vi "Agilent VNA Read Calibration Status.vi"(7 "Agilent VNA":T6, 8 "error in (no error)":errorcluster, 10 "Parameters to Measure":T2[](array[typedef]) {"Channel" min=1 max=99 step=1; "Parameter"."Stimulus Port" min=1 step=1; "Parameter"."Response Port" min=1 step=1}, 11 "VISA Resource Name":refnum<visa-resource-name>) -> (0 "error out":errorcluster {"code" format="%.0x"}, 1 "Parameters to Measure":T2[](array[typedef]) {"Channel" min=1 max=99 step=1; "Parameter"."Stimulus Port" min=1 step=1; "Parameter"."Response Port" min=1 step=1}, 2 "Calibration Type by Parameter":T1[](array[typedef]), 3 "dup VISA Resource Name":refnum<visa-resource-name>)   [LabVIEW 2011]
doc: "This VI for the HP 8753B is used to read the calibration type.\n\n0 response\n1 response and isolation\n2 S11 1-port\n3 S22 1-port\n4 full 2-port\n5 one path 2-port\n6 no cal detected"
uses:
  TypeDefs/Agilent VNA Instrument Info.ctl
  tests/S Parameter/TypeDefs/SP Parameter to Measure.ctl
  tests/S Parameter/TypeDefs/SP Parameter.ctl
  tests/S Parameter/TypeDefs/SP Calibration State.ctl
  tests/S Parameter/TypeDefs/SP Measurement Format.ctl
  TypeDefs/Agilent VNA Calibration State.ctl
  TypeDefs/Agilent VNA Measurement.ctl
  TypeDefs/Agilent VNA Conversion.ctl
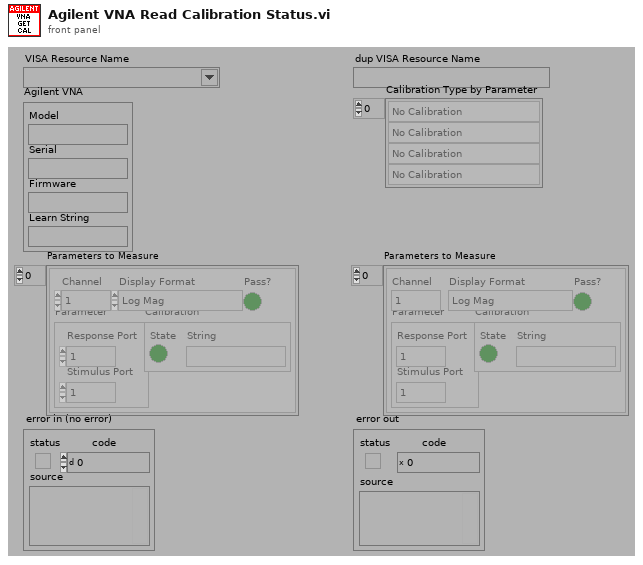
[diagram p1: front panel]
types:
  T1 = typedef "Agilent VNA Calibration State.ctl" = enum32{"No Calibration", "Response", "Response and Isolation", "Full 1-Port (Port 1)", "Full 1-Port (Port 2)", "Full 2-Port", "One Path 2-Port", "TRL/LRM  2-Port", "TOSM Multi-Port", "TOM 2-Port", "TRM 2-Port", "TNA 2-Port", "Full 1-Port (Port 3)", "Full 1-Port (Port 4)", "Full 3-Port", "Full 4-Port", "Full 1-Port (Port 5)", "Full 1-Port (Port 6)", "Full 1-Port (Port 7)", "Full 1-Port (Port 8)", "Full 5-Port", "Full 6-Port", "Full 7-Port", "Full 8-Port"}
  T2 = typedef "SP Parameter to Measure.ctl" = cluster{"Channel":i8, "Parameter":T3, "Calibration":T4, "Display Format":T5, "Pass?":bool}
  T3 = typedef "SP Parameter.ctl" = cluster{"Stimulus Port":i8, "Response Port":i8}
  T4 = typedef "SP Calibration State.ctl" = cluster{"State":bool, "String":string}
  T5 = typedef "SP Measurement Format.ctl" = enum32{"Log Mag", "Phase", "Delay", "Smith (R+jX)", "Polar (Re/Im)", "Linear Mag", "SWR", "Real", "Imaginary", "Smith (Lin/Phase)", "Smith (Log/Phase)", "Smith (Real/Imag)", "Smith (G+jB)", "Polar (Lin/Phase)", "Polar (Log/Phase)", "Expanded Phase", "Positive Phase", "Inverted Smith", "Unwrapped Phase", "Power Out", "Power In", "Linear Mag/Phase", "Log Mag/Phase", "Real/Imaginary"}
  T6 = typedef "Agilent VNA Instrument Info.ctl" = cluster{"Model":string, "Serial":string, "Firmware":string, "Learn String":string}
  T7 = typedef "Agilent VNA Model.ctl" = enum16{"Not Supported", "8510X", "8719X", "8720X", "8722X", "8753X", "ENA", "PNA", "Field Fox"}
  T8 = typedef "Agilent VNA Measurement.ctl" = enum32{"SXX", "Analog In - Aux In", "A/R", "B/R", "A/B", "A", "B", "R"}
  T9 = typedef "Agilent VNA Conversion.ctl" = enum16{"Off", "Z Reflection", "Z Transmit", "Y Reflection", "Y Transmit", "Inversion", "ZT Shunt", "YT Shunt", "Conjugation"}
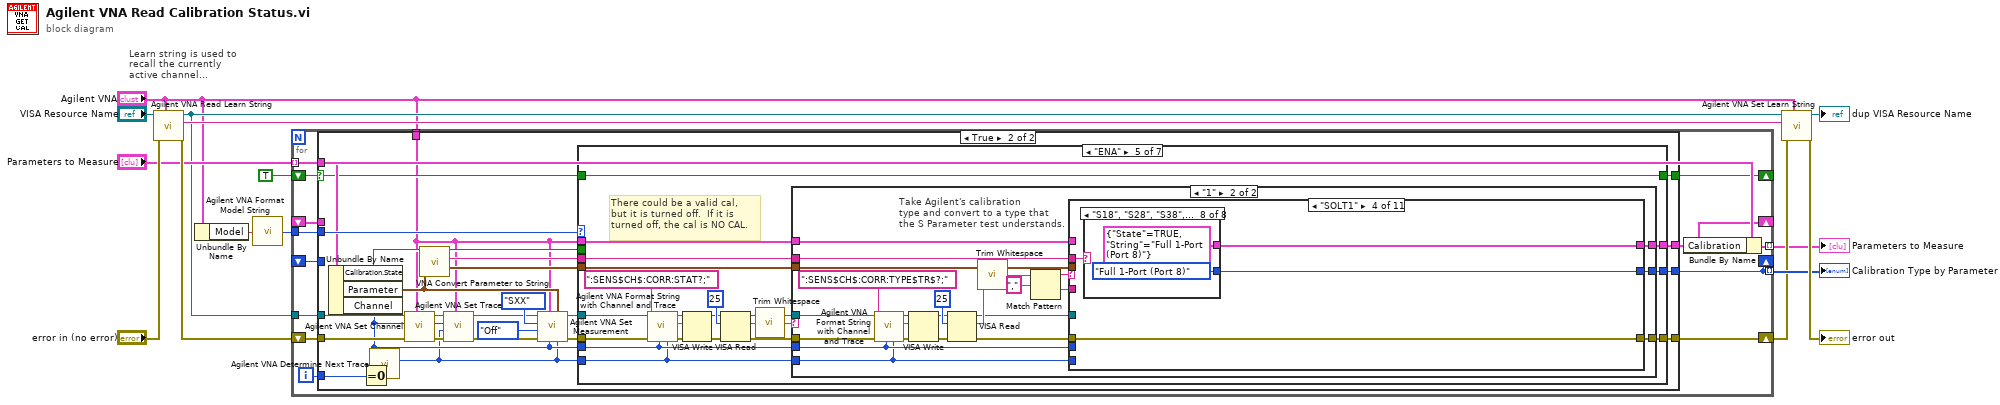
[diagram p0: block diagram]
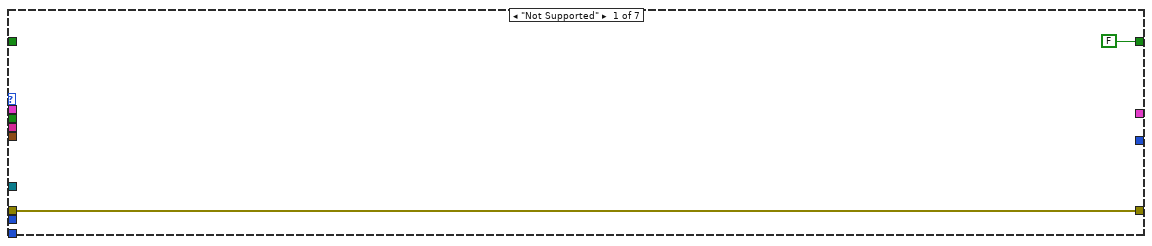
[diagram p3: hidden frame]
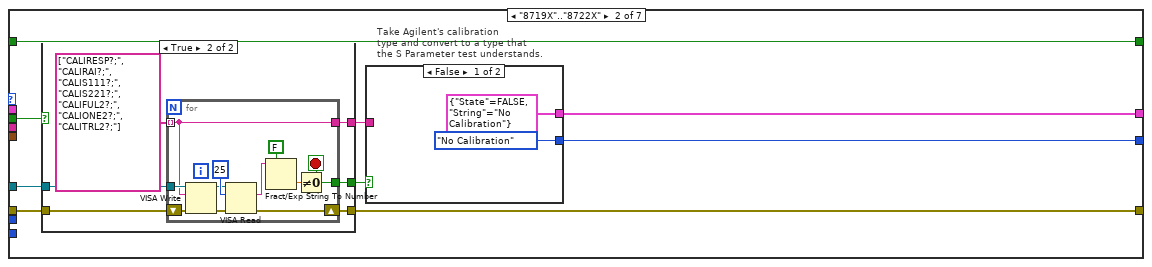
[diagram p4: hidden frame]
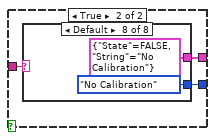
[diagram p6: hidden frame]
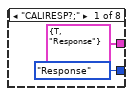
[diagram p7: hidden frame]
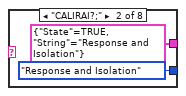
[diagram p8: hidden frame]
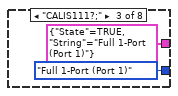
[diagram p9: hidden frame]
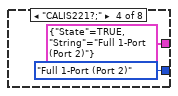
[diagram p10: hidden frame]
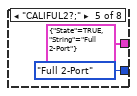
[diagram p11: hidden frame]
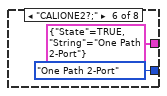
[diagram p12: hidden frame]
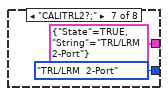
[diagram p13: hidden frame]
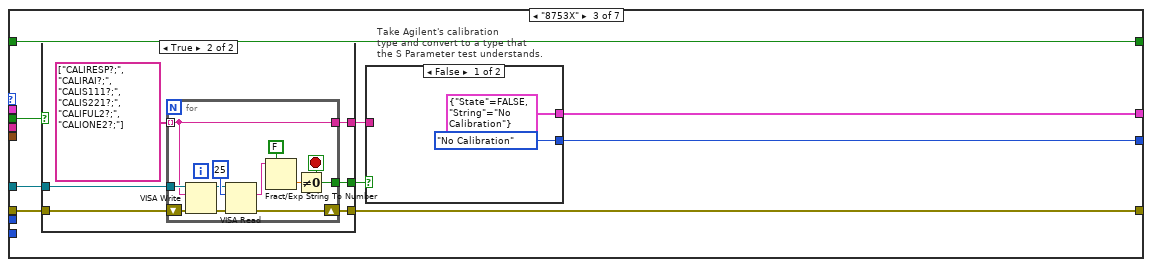
[diagram p14: hidden frame]
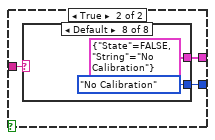
[diagram p16: hidden frame]
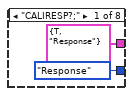
[diagram p17: hidden frame]
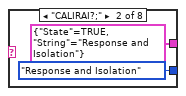
[diagram p18: hidden frame]
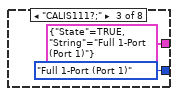
[diagram p19: hidden frame]
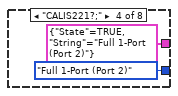
[diagram p20: hidden frame]
diagram:
  # "Learn string is used to\nrecall the currently \nactive channel..."
  n1 = call "Agilent VNA Read Learn String.vi"("Agilent VNA"="Agilent VNA", "error in (no error)"="error in (no error)", "VISA Resource Name"="VISA Resource Name") -> ("error out"=w8:errorcluster, "Learn String"=w13:string, "dup VISA Resource Name"=w6:refnum<visa-resource-name>)  [unwired: 6 out]
  n2 = Unbundle By Name("Agilent VNA") -> ("Model"=w4:string)
  n3 = call "Agilent VNA Format Model String.vi"("Model"=w4) -> ("Model"=w5:T7)
  n4 = for {
    tunnel: w6 -> [w28]
    shift-right: [w29] -> w9
    shift-left: w8 -> [w27]
    tunnel: "Parameters to Measure" -> [w24] mode=indexing
    tunnel: [w18] -> w10 mode=indexing
    tunnel: w5 -> [w25]
    tunnel: [w23] -> w3 mode=indexing
    shift-right: [w22] -> _
    shift-left: TRUE -> [w21]
    tunnel: "Agilent VNA" -> [w20]
    shift-right: [w19] -> _
    shift-left: _ -> [w16]
    shift-right: [w18] -> _
    shift-left: _ -> [w17]
    i -> [w26]
    n5 = case shown="True" w21 {
      selector: w21 -> [w32 w35]
      tunnel: [w33 w56] -> w29
      tunnel: w28 -> [_ w55]
      tunnel: w27 -> [w33 w54]
      tunnel: [w31 w50] -> w18
      tunnel: w26 -> [_ w41]
      tunnel: w25 -> [_ w39]
      tunnel: w24 -> [_ w38]
      tunnel: [w30 w37] -> w19
      tunnel: [w32 w36] -> w22
      tunnel: w20 -> [_ w34]
      tunnel: w17 -> [w31 _]
      tunnel: w16 -> [w30 _]
      frame False {
        # "Do not check subsequent channels and traces.\nJust duplicate the calibration."
      }
      frame True {
        n6 = Unbundle By Name(w38) -> ("Calibration.State"=w53:bool, "Parameter"=w48:T3, "Channel"=w43:i8)
        n7 = Equal To 0?(x=w41) -> (x = 0?=w40:bool)
        n8 = call "Agilent VNA Determine Next Trace.vi"("Reset?"=w40, "Channel"=w43) -> ("Next Trace"=w42:i8)  [unwired: 9 out]
        n9 = call "Agilent VNA Set Channel.vi"("Agilent VNA"=w34, "error in (no error)"=w54, "Channel"=w43, "VISA Resource Name"=w55) -> ("error out"=w47:errorcluster, "dup VISA Resource Name"=w46:refnum<visa-resource-name>)  [unwired: 6 out]
        n10 = call "VNA Convert Parameter to String.vi"("Parameter"=w48) -> ("Parameter String"=w51:string)  [unwired: 10 out]
        n11 = call "Agilent VNA Set Trace.vi"("Agilent VNA"=w34, "error in (no error)"=w47, "Trace"=w42, "Channel"=w43, "VISA Resource Name"=w46) -> ("error out"=w44:errorcluster, "dup VISA Resource Name"=w45:refnum<visa-resource-name>)  [unwired: 5 out]
        n12 = call "Agilent VNA Set Measurement.vi"("Trace"=w42, "Parameter"=w48, "Channel"=w43, "Agilent VNA"=w34, "error in (no error)"=w44, "Conversion (Off)"=Agilent_VNA_Conversion."Off", "Measurement (SXX)"=Agilent_VNA_Measurement."SXX" ("Measurement (S11 - A/R)"), "VISA Resource Name"=w45) -> ("error out"=w58:errorcluster, "dup VISA Resource Name"=w57:refnum<visa-resource-name>)  [unwired: 2 out]
        n13 = case shown="\"ENA\"" w39 {
          tunnel: w58 -> [w60 w69 w117 w174 w217 w344 w435]
          tunnel: w57 -> [_ w68 w116 w173 w212 w339 w433]
          tunnel: [w60 w67 w115 w169 w223 w349 w443] -> w56
          tunnel: [_ w66 w114 w167 w225 w351 w445] -> w50
          tunnel: w53 -> [_ w63 w111 _ _ _ _]
          tunnel: w43 -> [_ _ _ _ w210 w338 w429]
          tunnel: w51 -> [_ _ _ _ w224 w350 w444]
          tunnel: w34 -> [_ _ _ _ w222 w348 _]
          tunnel: [_ w62 w110 w159 w221 w347 w442] -> w37
          tunnel: w42 -> [_ _ _ _ w209 w337 w430]
          tunnel: w48 -> [_ _ _ _ w220 w346 _]
          tunnel: [FALSE w61 w109 w157 w206 FALSE w428] -> w36
          tunnel: w35 -> [_ w61 w109 w157 w206 _ w428]
          frame "Not Supported" {
          }
          frame "8719X".."8722X" {
            # "Take Agilent's calibration\ntype and convert to a type that\nthe S Parameter test understands."
            n14 = case shown="True" w63 {
              tunnel: w69 -> [w70 w76]
              tunnel: w68 -> [_ w75]
              tunnel: [w70 w74] -> w67
              tunnel: [_ w73] -> w65
              tunnel: [_ w72] -> w64
              frame False {
              }
              frame True {
                n15 = for {
                  tunnel: w75 -> [w86]
                  tunnel: [w77] -> w73
                  tunnel: [w78] -> w72
                  shift-right: [w85] -> w74
                  shift-left: w76 -> [w87]
                  tunnel: string[] ["CALIRESP?;", "CALIRAI?;", "CALIS111?;", "CALIS221?;", "CALIFUL2?;", "CALIONE2?;", "CALITRL2?;"] -> [w78] mode=indexing
                  stop <- w77 stop-if-true
                  n16 = VISA Write(VISA resource name=w86, write buffer=w78, error in (no error)=w87) -> (VISA resource name out=w80:refnum<visa-resource-name>, error out=w84:errorcluster)  [unwired: 1 out]
                  n17 = VISA Read(VISA resource name=w80, byte count=u32 25, error in (no error)=w84) -> (read buffer=w83:string, error out=w85:errorcluster)  [unwired: 2 out]
                  n18 = Fract/Exp String To Number(use system decimal point (T)=FALSE, string=w83) -> (number=w82:dbl)  [unwired: 3 out]
                  n19 = Not Equal To 0?(x=w82) -> (x != 0?=w77:bool)
                }
              }
            }
            n20 = case shown="False" w65 {
              tunnel: [Agilent_VNA_Calibration_State."No Calibration" ("S Parameter Test Cal Type") w92] -> w66
              tunnel: w64 -> [_ w91]
              tunnel: [T4 {"State"=FALSE, "String"="No Calibration"} w90] -> w62
              frame False {
              }
              frame True {
                n21 = case shown="Default" w91 {
                  tunnel: [Agilent_VNA_Calibration_State."Response" ("S Parameter Test Cal Type") Agilent_VNA_Calibration_State."Response and Isolation" ("S Parameter Test Cal Type") Agilent_VNA_Calibration_State."Full 1-Port (Port 1)" ("S Parameter Test Cal Type") Agilent_VNA_Calibration_State."Full 1-Port (Port 2)" ("S Parameter Test Cal Type") Agilent_VNA_Calibration_State."Full 2-Port" ("S Parameter Test Cal Type") Agilent_VNA_Calibration_State."One Path 2-Port" ("S Parameter Test Cal Type") Agilent_VNA_Calibration_State."TRL/LRM  2-Port" ("S Parameter Test Cal Type") Agilent_VNA_Calibration_State."No Calibration" ("S Parameter Test Cal Type")] -> w92
                  tunnel: [T4 {"State"=TRUE, "String"="Response"} T4 {"State"=TRUE, "String"="Response and Isolation"} T4 {"State"=TRUE, "String"="Full 1-Port (Port 1)"} T4 {"State"=TRUE, "String"="Full 1-Port (Port 2)"} T4 {"State"=TRUE, "String"="Full 2-Port"} T4 {"State"=TRUE, "String"="One Path 2-Port"} T4 {"State"=TRUE, "String"="TRL/LRM 2-Port"} T4 {"State"=FALSE, "String"="No Calibration"}] -> w90
                  frame "CALIRESP?;" {
                  }
                  frame "CALIRAI?;" {
                  }
                  frame "CALIS111?;" {
                  }
                  frame "CALIS221?;" {
                  }
                  frame "CALIFUL2?;" {
                  }
                  frame "CALIONE2?;" {
                  }
                  frame "CALITRL2?;" {
                  }
                  frame Default {
                  }
                }
              }
            }
          }
          frame "8753X" {
            # "Take Agilent's calibration\ntype and convert to a type that\nthe S Parameter test understands."
            n22 = case shown="True" w111 {
              tunnel: w117 -> [w118 w124]
              tunnel: w116 -> [_ w123]
              tunnel: [w118 w122] -> w115
              tunnel: [_ w121] -> w113
              tunnel: [_ w120] -> w112
              frame False {
              }
              frame True {
                n23 = for {
                  tunnel: w123 -> [w134]
                  tunnel: [w125] -> w121
                  tunnel: [w126] -> w120
                  shift-right: [w133] -> w122
                  shift-left: w124 -> [w135]
                  tunnel: string[] ["CALIRESP?;", "CALIRAI?;", "CALIS111?;", "CALIS221?;", "CALIFUL2?;", "CALIONE2?;"] -> [w126] mode=indexing
                  stop <- w125 stop-if-true
                  n24 = VISA Write(VISA resource name=w134, write buffer=w126, error in (no error)=w135) -> (VISA resource name out=w128:refnum<visa-resource-name>, error out=w132:errorcluster)  [unwired: 1 out]
                  n25 = VISA Read(VISA resource name=w128, byte count=u32 25, error in (no error)=w132) -> (read buffer=w131:string, error out=w133:errorcluster)  [unwired: 2 out]
                  n26 = Fract/Exp String To Number(use system decimal point (T)=FALSE, string=w131) -> (number=w130:dbl)  [unwired: 3 out]
                  n27 = Not Equal To 0?(x=w130) -> (x != 0?=w125:bool)
                }
              }
            }
            n28 = case shown="False" w113 {
              tunnel: [Agilent_VNA_Calibration_State."No Calibration" ("S Parameter Test Cal Type") w140] -> w114
              tunnel: w112 -> [_ w139]
              tunnel: [T4 {"State"=FALSE, "String"="No Calibration"} w138] -> w110
              frame False {
              }
              frame True {
                n29 = case shown="Default" w139 {
                  tunnel: [Agilent_VNA_Calibration_State."Response" ("S Parameter Test Cal Type") Agilent_VNA_Calibration_State."Response and Isolation" ("S Parameter Test Cal Type") Agilent_VNA_Calibration_State."Full 1-Port (Port 1)" ("S Parameter Test Cal Type") Agilent_VNA_Calibration_State."Full 1-Port (Port 2)" ("S Parameter Test Cal Type") Agilent_VNA_Calibration_State."Full 2-Port" ("S Parameter Test Cal Type") Agilent_VNA_Calibration_State."One Path 2-Port" ("S Parameter Test Cal Type") Agilent_VNA_Calibration_State."TRL/LRM  2-Port" ("S Parameter Test Cal Type") Agilent_VNA_Calibration_State."No Calibration" ("S Parameter Test Cal Type")] -> w140
                  tunnel: [T4 {"State"=TRUE, "String"="Response"} T4 {"State"=TRUE, "String"="Response and Isolation"} T4 {"State"=TRUE, "String"="Full 1-Port (Port 1)"} T4 {"State"=TRUE, "String"="Full 1-Port (Port 2)"} T4 {"State"=TRUE, "String"="Full 2-Port"} T4 {"State"=TRUE, "String"="One Path 2-Port"} T4 {"State"=TRUE, "String"="TRL/LRM 2-Port"} T4 {"State"=FALSE, "String"="No Calibration"}] -> w138
                  frame "CALIRESP?;" {
                  }
                  frame "CALIRAI?;" {
                  }
                  frame "CALIS111?;" {
                  }
                  frame "CALIS221?;" {
                  }
                  frame "CALIFUL2?;" {
                  }
                  frame "CALIONE2?;" {
                  }
                  frame "CALITRL2?;" {
                  }
                  frame Default {
                  }
                }
              }
            }
          }
          frame "8510X" {
            # "Take Agilent's calibration\ntype and convert to a type that\nthe S Parameter test understands."
            n30 = VISA Write(VISA resource name=w173, write buffer="CALI?;", error in (no error)=w174) -> (VISA resource name out=w164:refnum<visa-resource-name>, error out=w166:errorcluster)  [unwired: 1 out]
            n31 = VISA Read(VISA resource name=w164, byte count=u32 25, error in (no error)=w166) -> (VISA resource name out=w171:refnum<visa-resource-name>, read buffer=w162:string, error out=w170:errorcluster)  [unwired: 1 out]
            n32 = call <vilib>:"Trim Whitespace.vi"("string"=w162) -> ("trimmed string"=w161:string)  [unwired: 1 in]
            n33 = call "Strip Quotes From String.vi"("String In"=w161) -> ("Trimmed String"=w172:string)
            n34 = case shown="\"RECEIVER\", \"UNDEFINED\", Default" w172 {
              tunnel: [Agilent_VNA_Calibration_State."Response" ("S Parameter Test Cal Type") Agilent_VNA_Calibration_State."Response and Isolation" ("S Parameter Test Cal Type") Agilent_VNA_Calibration_State."Full 1-Port (Port 1)" ("S Parameter Test Cal Type") Agilent_VNA_Calibration_State."Full 1-Port (Port 2)" ("S Parameter Test Cal Type") Agilent_VNA_Calibration_State."Full 2-Port" ("S Parameter Test Cal Type") Agilent_VNA_Calibration_State."TRL/LRM  2-Port" ("S Parameter Test Cal Type") Agilent_VNA_Calibration_State."No Calibration" ("S Parameter Test Cal Type") Agilent_VNA_Calibration_State."One Path 2-Port" ("S Parameter Test Cal Type")] -> w160
              tunnel: [T4 {"State"=TRUE, "String"="Response"} T4 {"State"=TRUE, "String"="Response and Isolation"} T4 {"State"=TRUE, "String"="Full 1-Port (Port 1)"} T4 {"State"=TRUE, "String"="Full 1-Port (Port 2)"} T4 {"State"=TRUE, "String"="Full 2-Port"} T4 {"State"=TRUE, "String"="TRL/LRM 2-Port"} T4 {"State"=FALSE, "String"="No Calibration"} T4 {"State"=TRUE, "String"="One Path 2-Port"}] -> w158
              frame "RESPONSE" {
              }
              frame "RESPONSE  & ISOL'N" {
              }
              frame "S11 1-PORT" {
              }
              frame "S22 1-PORT" {
              }
              frame "2-PORT" {
              }
              frame "CALITRL2?;" {
              }
              frame "RECEIVER", "UNDEFINED", Default {
              }
              frame "ONE PATH 2-PORT" {
              }
            }
            n35 = case shown="\"No Calibration\"" w160 {
              tunnel: w170 -> [w179 w189]
              tunnel: w171 -> [_ w188]
              tunnel: [w179 w187] -> w169
              tunnel: [_ w180] -> w168
              frame Default {
              }
              frame "No Calibration" {
                n36 = VISA Write(VISA resource name=w188, write buffer="CALZ?;", error in (no error)=w189) -> (VISA resource name out=w184:refnum<visa-resource-name>, error out=w186:errorcluster)  [unwired: 1 out]
                n37 = VISA Read(VISA resource name=w184, byte count=u32 25, error in (no error)=w186) -> (read buffer=w181:string, error out=w187:errorcluster)  [unwired: 2 out]
                n38 = call <vilib>:"Trim Whitespace.vi"("string"=w181) -> ("trimmed string"=w182:string)  [unwired: 1 in]
                n39 = call "Strip Quotes From String.vi"("String In"=w182) -> ("Trimmed String"=w180:string)
              }
            }
            n40 = case shown="\"CALITRL2?;\", \"LINE Z0\", \"SYSTEM\", \"THRU\"" w168 {
              tunnel: [Agilent_VNA_Calibration_State."TRL/LRM  2-Port" ("S Parameter Test Cal Type") w178] -> w167
              tunnel: w160 -> [_ w178]
              tunnel: [T4 {"State"=TRUE, "String"="TRL/LRM 2-Port"} w177] -> w159
              tunnel: w158 -> [_ w177]
              frame "CALITRL2?;", "LINE Z0", "SYSTEM", "THRU" {
              }
              frame Default {
              }
            }
          }
          frame "ENA" {
            # "There could be a valid cal,\nbut it is turned off.  If it is\nturned off, the cal is NO CAL."
            n41 = call "Agilent VNA Format String with Channel and Trace.vi"("Trace"=w209, "Channel"=w210, "String"=":SENS$CH$:CORR:STAT?;") -> ("String Out"=w219:string)  [unwired: 6 out]
            n42 = VISA Write(VISA resource name=w212, write buffer=w219, error in (no error)=w217) -> (VISA resource name out=w213:refnum<visa-resource-name>, error out=w216:errorcluster)  [unwired: 1 out]
            n43 = VISA Read(VISA resource name=w213, byte count=u32 25, error in (no error)=w216) -> (VISA resource name out=w214:refnum<visa-resource-name>, read buffer=w208:string, error out=w215:errorcluster)  [unwired: 1 out]
            n44 = call <vilib>:"Trim Whitespace.vi"("string"=w208) -> ("trimmed string"=w207:string)  [unwired: 1 in]
            n45 = case shown="\"1\"" w207 {
              tunnel: [Agilent_VNA_Calibration_State."No Calibration" ("S Parameter Test Cal Type") w250] -> w225
              tunnel: w215 -> [w226 w244]
              tunnel: w214 -> [_ w243]
              tunnel: w224 -> [_ w235]
              tunnel: [w226 w234] -> w223
              tunnel: w222 -> [_ w233]
              tunnel: [T4 {"State"=FALSE, "String"="No Calibration"} w232] -> w221
              tunnel: w210 -> [_ w231]
              tunnel: w209 -> [_ w230]
              tunnel: w220 -> [_ w229]
              frame "0", Default {
              }
              frame "1" {
                # "Take Agilent's calibration\ntype and convert to a type that\nthe S Parameter test understands."
                n46 = call "Agilent VNA Format String with Channel and Trace.vi"("Trace"=w230, "Channel"=w231, "String"=":SENS$CH$:CORR:TYPE$TR$?;") -> ("String Out"=w247:string)  [unwired: 6 out]
                n47 = VISA Write(VISA resource name=w243, write buffer=w247, error in (no error)=w244) -> (VISA resource name out=w248:refnum<visa-resource-name>, error out=w242:errorcluster)  [unwired: 1 out]
                n48 = VISA Read(VISA resource name=w248, byte count=u32 25, error in (no error)=w242) -> (VISA resource name out=w236:refnum<visa-resource-name>, read buffer=w245:string, error out=w237:errorcluster)  [unwired: 1 out]
                n49 = call <vilib>:"Trim Whitespace.vi"("string"=w245) -> ("trimmed string"=w241:string)  [unwired: 1 in]
                n50 = Match Pattern(string=w241, regular expression=",") -> (before substring=w240:string, after substring=w238:string)  [unwired: 3 out]
                n51 = case shown="\"SOLT1\"" w240 {
                  tunnel: [Agilent_VNA_Calibration_State."No Calibration" ("S Parameter Test Cal Type") Agilent_VNA_Calibration_State."Response" ("S Parameter Test Cal Type") w287 w295 Agilent_VNA_Calibration_State."Full 2-Port" ("S Parameter Test Cal Type") Agilent_VNA_Calibration_State."Full 3-Port" ("S Parameter Test Cal Type") Agilent_VNA_Calibration_State."Full 4-Port" ("S Parameter Test Cal Type") Agilent_VNA_Calibration_State."Full 5-Port" ("S Parameter Test Cal Type") Agilent_VNA_Calibration_State."Full 6-Port" ("S Parameter Test Cal Type") Agilent_VNA_Calibration_State."Full 7-Port" ("S Parameter Test Cal Type") Agilent_VNA_Calibration_State."Full 8-Port" ("S Parameter Test Cal Type")] -> w250
                  tunnel: w238 -> [_ _ _ _ _ _ _ _ _ _ _]
                  tunnel: w237 -> [w252 w255 w282 w294 w313 w316 w319 w322 w325 w328 w331]
                  tunnel: w231 -> [_ _ w263 _ _ _ _ _ _ _ _]
                  tunnel: [w252 w255 w284 w294 w313 w316 w319 w322 w325 w328 w331] -> w234
                  tunnel: w236 -> [_ _ w281 _ _ _ _ _ _ _ _]
                  tunnel: w233 -> [_ _ w278 _ _ _ _ _ _ _ _]
                  tunnel: w235 -> [_ _ _ w293 _ _ _ _ _ _ _]
                  tunnel: [T4 {"State"=FALSE, "String"="No Calibration"} T4 {"State"=TRUE, "String"="Response"} w264 w292 T4 {"State"=TRUE, "String"="Full 2-Port"} T4 {"State"=TRUE, "String"="Full 3-Port"} T4 {"State"=TRUE, "String"="Full 4-Port"} T4 {"State"=TRUE, "String"="Full 5-Port"} T4 {"State"=TRUE, "String"="Full 6-Port"} T4 {"State"=TRUE, "String"="Full 7-Port"} T4 {"State"=TRUE, "String"="Full 8-Port"}] -> w232
                  tunnel: w230 -> [_ _ w262 _ _ _ _ _ _ _ _]
                  tunnel: w229 -> [_ _ w261 _ _ _ _ _ _ _ _]
                  frame "NONE", Default {
                  }
                  frame "RESPO", "RESPS" {
                  }
                  frame "ERES", "RESPT" {
                    n52 = call "Agilent VNA Read Number of Points.vi"("Channel"=w263, "Agilent VNA"=w278, "error in (no error)"=w282, "VISA Resource Name"=w281) -> ("error out"=w279:errorcluster, "Number Points"=w277:i32, "dup VISA Resource Name"=w280:refnum<visa-resource-name>)  [unwired: 5 out]
                    n53 = Unbundle By Name(w261) -> ("Response Port"=w260:i8, "Stimulus Port"=w259:i8)
                    n54 = Multiply(x=u32 40 ("byte count"), y=w277) -> (x*y=w275:u32)
                    n55 = Format Into String(format string=":SENS$CH$:CORR:COEF? EX,%d,%d;" ("String"), w260, w259) -> (resulting string=w257:string)  [unwired: 2 in, 1 out]
                    n56 = call "Agilent VNA Format String with Channel and Trace.vi"("Trace"=w262, "Channel"=w263, "String"=w257) -> ("String Out"=w286:string)  [unwired: 6 out]
                    n57 = VISA Write(VISA resource name=w280, write buffer=w286, error in (no error)=w279) -> (VISA resource name out=w283:refnum<visa-resource-name>, error out=w285:errorcluster)  [unwired: 1 out]
                    n58 = VISA Read(VISA resource name=w283, byte count=w275, error in (no error)=w285) -> (read buffer=w272:string, error out=w284:errorcluster)  [unwired: 2 out]
                    n59 = Spreadsheet String To Array(delimiter (Tab)=",", format string="%f", spreadsheet string=w272, array type (2D Dbl)=dbl[] []) -> (array=w270:dbl[])
                    n60 = Array Max & Min(array=w270) -> (max value=w269:dbl, min value=w266:dbl)  [unwired: 2 out]
                    n61 = Equal To 0?(x=w269) -> (x = 0?=w267:bool)
                    n62 = Equal To 0?(x=w266) -> (x = 0?=w265:bool)
                    n63 = And(x=w267, y=w265) -> (x .and. y?=w268:bool)
                    n64 = case shown="False" w268 {
                      tunnel: [Agilent_VNA_Calibration_State."Response" ("S Parameter Test Cal Type") Agilent_VNA_Calibration_State."Response and Isolation" ("S Parameter Test Cal Type")] -> w287
                      tunnel: [T4 {"State"=TRUE, "String"="Response"} T4 {"State"=TRUE, "String"="Response and Isolation"}] -> w264
                      frame True {
                      }
                      frame False {
                      }
                    }
                  }
                  frame "SOLT1" {
                    n65 = case shown="\"S18\", \"S28\", \"S38\", \"S48\", \"S58\", \"S68\", \"S78\", \"S88\"" w293 {
                      tunnel: [Agilent_VNA_Calibration_State."Full 1-Port (Port 1)" ("S Parameter Test Cal Type") Agilent_VNA_Calibration_State."Full 1-Port (Port 2)" ("S Parameter Test Cal Type") Agilent_VNA_Calibration_State."Full 1-Port (Port 3)" ("S Parameter Test Cal Type") Agilent_VNA_Calibration_State."Full 1-Port (Port 4)" ("S Parameter Test Cal Type") Agilent_VNA_Calibration_State."Full 1-Port (Port 5)" ("S Parameter Test Cal Type") Agilent_VNA_Calibration_State."Full 1-Port (Port 6)" ("S Parameter Test Cal Type") Agilent_VNA_Calibration_State."Full 1-Port (Port 7)" ("S Parameter Test Cal Type") Agilent_VNA_Calibration_State."Full 1-Port (Port 8)" ("S Parameter Test Cal Type")] -> w295
                      tunnel: [T4 {"State"=TRUE, "String"="Full 1-Port (Port 1)"} T4 {"State"=TRUE, "String"="Full 1-Port (Port 2)"} T4 {"State"=TRUE, "String"="Full 1-Port (Port 3)"} T4 {"State"=TRUE, "String"="Full 1-Port (Port 4)"} T4 {"State"=TRUE, "String"="Full 1-Port (Port 5)"} T4 {"State"=TRUE, "String"="Full 1-Port (Port 6)"} T4 {"State"=TRUE, "String"="Full 1-Port (Port 7)"} T4 {"State"=TRUE, "String"="Full 1-Port (Port 8)"}] -> w292
                      frame "S11", "S21", "S31", "S41", "S51", "S61", "S71", "S81", Default {
                      }
                      frame "S12", "S22", "S32", "S42", "S52", "S62", "S72", "S82" {
                      }
                      frame "S13", "S23", "S33", "S43", "S53", "S63", "S73", "S83" {
                      }
                      frame "S14", "S24", "S34", "S44", "S54", "S64", "S74", "S84" {
                      }
                      frame "S15", "S25", "S35", "S45", "S55", "S65", "S75", "S85" {
                      }
                      frame "S16", "S26", "S36", "S46", "S56", "S66", "S76", "S86" {
                      }
                      frame "S17", "S27", "S37", "S47", "S57", "S67", "S77", "S87" {
                      }
                      frame "S18", "S28", "S38", "S48", "S58", "S68", "S78", "S88" {
                      }
                    }
                  }
                  frame "SOLT2" {
                  }
                  frame "SOLT3" {
                  }
                  frame "SOLT4" {
                  }
                  frame "SOLT5" {
                  }
                  frame "SOLT6" {
                  }
                  frame "SOLT7" {
                  }
                  frame "SOLT8" {
                  }
                }
              }
            }
          }
          frame "Field Fox" {
            # "There could be a valid cal,\nbut it is turned off.  If it is\nturned off, the cal is NO CAL."
            n66 = VISA Write(VISA resource name=w339, write buffer=":SENS:CORR:STAT?;", error in (no error)=w344) -> (VISA resource name out=w340:refnum<visa-resource-name>, error out=w343:errorcluster)  [unwired: 1 out]
            n67 = VISA Read(VISA resource name=w340, byte count=u32 25, error in (no error)=w343) -> (VISA resource name out=w341:refnum<visa-resource-name>, read buffer=w336:string, error out=w342:errorcluster)  [unwired: 1 out]
            n68 = call <vilib>:"Trim Whitespace.vi"("string"=w336) -> ("trimmed string"=w335:string)  [unwired: 1 in]
            n69 = case shown="\"1\"" w335 {
              tunnel: [Agilent_VNA_Calibration_State."No Calibration" ("S Parameter Test Cal Type") w375] -> w351
              tunnel: w342 -> [w352 w371]
              tunnel: w341 -> [_ w370]
              tunnel: w350 -> [_ w362]
              tunnel: [w352 w361] -> w349
              tunnel: w348 -> [_ w360]
              tunnel: [T4 {"State"=FALSE, "String"="No Calibration"} w359] -> w347
              tunnel: w338 -> [_ w358]
              tunnel: w337 -> [_ w357]
              tunnel: w346 -> [_ w356]
              frame "0", Default {
              }
              frame "1" {
                # "Take Agilent's calibration\ntype and convert to a type that\nthe S Parameter test understands."
                n70 = VISA Write(VISA resource name=w370, write buffer=":SENS:CORR:COLL:METH:TYPE?;" ("String"), error in (no error)=w371) -> (VISA resource name out=w373:refnum<visa-resource-name>, error out=w369:errorcluster)  [unwired: 1 out]
                n71 = VISA Read(VISA resource name=w373, byte count=u32 25, error in (no error)=w369) -> (VISA resource name out=w363:refnum<visa-resource-name>, read buffer=w372:string, error out=w364:errorcluster)  [unwired: 1 out]
                n72 = call <vilib>:"Trim Whitespace.vi"("string"=w372) -> ("trimmed string"=w368:string)  [unwired: 1 in]
                n73 = Match Pattern(string=w368, regular expression=",") -> (before substring=w367:string, after substring=w365:string)  [unwired: 3 out]
                n74 = case shown="\"RESPO\", \"RESPS\"" w367 {
                  tunnel: [Agilent_VNA_Calibration_State."No Calibration" ("S Parameter Test Cal Type") Agilent_VNA_Calibration_State."Response" ("S Parameter Test Cal Type") w412 w420 Agilent_VNA_Calibration_State."Full 2-Port" ("S Parameter Test Cal Type")] -> w375
                  tunnel: w365 -> [_ _ _ _ _]
                  tunnel: w364 -> [w377 w380 w407 w419 w426]
                  tunnel: w358 -> [_ _ w388 _ _]
                  tunnel: [w377 w380 w409 w419 w426] -> w361
                  tunnel: w363 -> [_ _ w406 _ _]
                  tunnel: w360 -> [_ _ w403 _ _]
                  tunnel: w362 -> [_ _ _ w418 _]
                  tunnel: [T4 {"State"=FALSE, "String"="No Calibration"} T4 {"State"=TRUE, "String"="Response"} w389 w417 T4 {"State"=TRUE, "String"="Full 2-Port"}] -> w359
                  tunnel: w357 -> [_ _ w387 _ _]
                  tunnel: w356 -> [_ _ w386 _ _]
                  frame "NONE", Default {
                  }
                  frame "RESPO", "RESPS" {
                  }
                  frame "ERES", "RESPT" {
                    n75 = call "Agilent VNA Read Number of Points.vi"("Channel"=w388, "Agilent VNA"=w403, "error in (no error)"=w407, "VISA Resource Name"=w406) -> ("error out"=w404:errorcluster, "Number Points"=w402:i32, "dup VISA Resource Name"=w405:refnum<visa-resource-name>)  [unwired: 5 out]
                    n76 = Unbundle By Name(w386) -> ("Response Port"=w385:i8, "Stimulus Port"=w384:i8)
                    n77 = Multiply(x=u32 40 ("byte count"), y=w402) -> (x*y=w400:u32)
                    n78 = Format Into String(format string=":SENS:CORR:COEF? EX,%d,%d;" ("String"), w385, w384) -> (resulting string=w382:string)  [unwired: 2 in, 1 out]
                    n79 = call "Agilent VNA Format String with Channel and Trace.vi"("Trace"=w387, "Channel"=w388, "String"=w382) -> ("String Out"=w411:string)  [unwired: 6 out]
                    n80 = VISA Write(VISA resource name=w405, write buffer=w411, error in (no error)=w404) -> (VISA resource name out=w408:refnum<visa-resource-name>, error out=w410:errorcluster)  [unwired: 1 out]
                    n81 = VISA Read(VISA resource name=w408, byte count=w400, error in (no error)=w410) -> (read buffer=w397:string, error out=w409:errorcluster)  [unwired: 2 out]
                    n82 = Spreadsheet String To Array(delimiter (Tab)=",", format string="%f", spreadsheet string=w397, array type (2D Dbl)=dbl[] []) -> (array=w395:dbl[])
                    n83 = Array Max & Min(array=w395) -> (max value=w394:dbl, min value=w391:dbl)  [unwired: 2 out]
                    n84 = Equal To 0?(x=w394) -> (x = 0?=w392:bool)
                    n85 = Equal To 0?(x=w391) -> (x = 0?=w390:bool)
                    n86 = And(x=w392, y=w390) -> (x .and. y?=w393:bool)
                    n87 = case shown="False" w393 {
                      tunnel: [Agilent_VNA_Calibration_State."Response" ("S Parameter Test Cal Type") Agilent_VNA_Calibration_State."Response and Isolation" ("S Parameter Test Cal Type")] -> w412
                      tunnel: [T4 {"State"=TRUE, "String"="Response"} T4 {"State"=TRUE, "String"="Response and Isolation"}] -> w389
                      frame True {
                      }
                      frame False {
                      }
                    }
                  }
                  frame "SOLT1" {
                    n88 = case shown="\"S12\", \"S22\"" w418 {
                      tunnel: [Agilent_VNA_Calibration_State."Full 1-Port (Port 1)" ("S Parameter Test Cal Type") Agilent_VNA_Calibration_State."Full 1-Port (Port 2)" ("S Parameter Test Cal Type")] -> w420
                      tunnel: [T4 {"State"=TRUE, "String"="Full 1-Port (Port 1)"} T4 {"State"=TRUE, "String"="Full 1-Port (Port 2)"}] -> w417
                      frame "S11", "S21", Default {
                      }
                      frame "S12", "S22" {
                      }
                    }
                  }
                  frame "SOLT2" {
                  }
                }
              }
            }
          }
          frame "PNA" {
            # "There could be a valid cal,\nbut it is turned off.  If it is\nturned off, the cal is NO CAL."
            n89 = call "Agilent VNA Format String with Channel and Trace.vi"("Trace"=w430, "Channel"=w429, "String"=":SENS$CH$:CORR:STAT?;") -> ("String Out"=w441:string)  [unwired: 6 out]
            n90 = VISA Write(VISA resource name=w433, write buffer=w441, error in (no error)=w435) -> (VISA resource name out=w438:refnum<visa-resource-name>, error out=w439:errorcluster)  [unwired: 1 out]
            n91 = VISA Read(VISA resource name=w438, byte count=u32 25, error in (no error)=w439) -> (VISA resource name out=w432:refnum<visa-resource-name>, read buffer=w436:string, error out=w434:errorcluster)  [unwired: 1 out]
            n92 = call <vilib>:"Trim Whitespace.vi"("string"=w436) -> ("trimmed string"=w431:string)  [unwired: 1 in]
            n93 = case shown="\"1\"" w431 {
              tunnel: [Agilent_VNA_Calibration_State."No Calibration" ("S Parameter Test Cal Type") w465] -> w445
              tunnel: w434 -> [w448 w460]
              tunnel: w432 -> [_ w459]
              tunnel: w444 -> [_ w457]
              tunnel: [w448 w452] -> w443
              tunnel: [T4 {"State"=FALSE, "String"="No Calibration"} w451] -> w442
              tunnel: w429 -> [_ w450]
              tunnel: w430 -> [_ w449]
              frame "0", Default {
              }
              frame "1" {
                # "Take Agilent's calibration\ntype and convert to a type that\nthe S Parameter test understands."
                n94 = call "Agilent VNA Format String with Channel and Trace.vi"("Trace"=w449, "Channel"=w450, "String"=":CALC$CH$:CORR:TYPE?;") -> ("String Out"=w462:string)  [unwired: 6 out]
                n95 = VISA Write(VISA resource name=w459, write buffer=w462, error in (no error)=w460) -> (VISA resource name out=w463:refnum<visa-resource-name>, error out=w458:errorcluster)  [unwired: 1 out]
                n96 = VISA Read(VISA resource name=w463, byte count=u32 50, error in (no error)=w458) -> (read buffer=w455:string, error out=w452:errorcluster)  [unwired: 2 out]
                n97 = Scan From String(format string="\"%[^(](%[^)]", input string=w455) -> (output 1=w454:string, output 2=w453:string)  [unwired: 2 in, 5 out]
                n98 = case shown="\"Full 1 Port\"" w454 {
                  tunnel: [Agilent_VNA_Calibration_State."No Calibration" ("S Parameter Test Cal Type") w470 Agilent_VNA_Calibration_State."Full 2-Port" ("S Parameter Test Cal Type") Agilent_VNA_Calibration_State."Full 3-Port" ("S Parameter Test Cal Type") Agilent_VNA_Calibration_State."Full 4-Port" ("S Parameter Test Cal Type") Agilent_VNA_Calibration_State."Full 5-Port" ("S Parameter Test Cal Type") Agilent_VNA_Calibration_State."Full 6-Port" ("S Parameter Test Cal Type") Agilent_VNA_Calibration_State."Full 7-Port" ("S Parameter Test Cal Type") Agilent_VNA_Calibration_State."Full 8-Port" ("S Parameter Test Cal Type") w507 w517] -> w465
                  tunnel: w457 -> [_ _ _ _ _ _ _ _ _ w511 w521]
                  tunnel: w453 -> [_ w469 _ _ _ _ _ _ _ w512 w522]
                  tunnel: [T4 {"State"=FALSE, "String"="No Calibration"} w468 T4 {"State"=TRUE, "String"="Full 2-Port"} T4 {"State"=TRUE, "String"="Full 3-Port"} T4 {"State"=TRUE, "String"="Full 4-Port"} T4 {"State"=TRUE, "String"="Full 5-Port"} T4 {"State"=TRUE, "String"="Full 6-Port"} T4 {"State"=TRUE, "String"="Full 7-Port"} T4 {"State"=TRUE, "String"="Full 8-Port"} w505 w515] -> w451
                  frame Default {
                  }
                  frame "Full 1 Port" {
                    n99 = case shown="\"8\"" w469 {
                      tunnel: [Agilent_VNA_Calibration_State."No Calibration" ("S Parameter Test Cal Type") Agilent_VNA_Calibration_State."Full 1-Port (Port 1)" ("S Parameter Test Cal Type") Agilent_VNA_Calibration_State."Full 1-Port (Port 2)" ("S Parameter Test Cal Type") Agilent_VNA_Calibration_State."Full 1-Port (Port 3)" ("S Parameter Test Cal Type") Agilent_VNA_Calibration_State."Full 1-Port (Port 4)" ("S Parameter Test Cal Type") Agilent_VNA_Calibration_State."Full 1-Port (Port 5)" ("S Parameter Test Cal Type") Agilent_VNA_Calibration_State."Full 1-Port (Port 6)" ("S Parameter Test Cal Type") Agilent_VNA_Calibration_State."Full 1-Port (Port 7)" ("S Parameter Test Cal Type") Agilent_VNA_Calibration_State."Full 1-Port (Port 8)" ("S Parameter Test Cal Type")] -> w470
                      tunnel: [T4 {"State"=FALSE, "String"="No Calibration"} T4 {"State"=TRUE, "String"="Full 1-Port (Port 1)"} T4 {"State"=TRUE, "String"="Full 1-Port (Port 2)"} T4 {"State"=TRUE, "String"="Full 1-Port (Port 3)"} T4 {"State"=TRUE, "String"="Full 1-Port (Port 4)"} T4 {"State"=TRUE, "String"="Full 1-Port (Port 5)"} T4 {"State"=TRUE, "String"="Full 1-Port (Port 6)"} T4 {"State"=TRUE, "String"="Full 1-Port (Port 7)"} T4 {"State"=TRUE, "String"="Full 1-Port (Port 8)"}] -> w468
                      frame Default {
                      }
                      frame "1" {
                      }
                      frame "2" {
                      }
                      frame "3" {
                      }
                      frame "4" {
                      }
                      frame "5" {
                      }
                      frame "6" {
                      }
                      frame "7" {
                      }
                      frame "8" {
                      }
                    }
                  }
                  frame "Full 2 Port" {
                  }
                  frame "Full 3 Port" {
                  }
                  frame "Full 4 Port" {
                  }
                  frame "Full 5 Port" {
                  }
                  frame "Full 6 Port" {
                  }
                  frame "Full 7 Port" {
                  }
                  frame "Full 8 Port" {
                  }
                  frame "Response" {
                    n100 = Format Into String(w511) -> (resulting string=w510:string)  [unwired: 3 in, 1 out]
                    n101 = Equal?(x=w510, y=w512) -> (x = y?=w503:bool)
                    n102 = Select(t=Agilent_VNA_Calibration_State."Response" ("S Parameter Test Cal Type"), s=w503, f=Agilent_VNA_Calibration_State."No Calibration") -> (s? t:f=w507:T1)
                    n103 = Format Into String(w507) -> (resulting string=w504:string)  [unwired: 3 in, 1 out]
                    n104 = Bundle By Name(cluster=T4 {"State"=FALSE, "String"=""}, "State"=w503, "String"=w504) -> (w505:T4)
                  }
                  frame "ResponseAndIsolation" {
                    n105 = Format Into String(w521) -> (resulting string=w520:string)  [unwired: 3 in, 1 out]
                    n106 = Equal?(x=w520, y=w522) -> (x = y?=w513:bool)
                    n107 = Select(t=Agilent_VNA_Calibration_State."Response and Isolation" ("S Parameter Test Cal Type"), s=w513, f=Agilent_VNA_Calibration_State."No Calibration") -> (s? t:f=w517:T1)
                    n108 = Format Into String(w517) -> (resulting string=w514:string)  [unwired: 3 in, 1 out]
                    n109 = Bundle By Name(cluster=T4 {"State"=FALSE, "String"=""}, "State"=w513, "String"=w514) -> (w515:T4)
                  }
                }
              }
            }
          }
        }
      }
    }
    n110 = Bundle By Name(cluster=w24, "Calibration"=w19) -> (w23:T2)
  }
  "Parameters to Measure" <- w3
  "Calibration Type by Parameter" <- w10
  n111 = call "Agilent VNA Set Learn String.vi"("Agilent VNA"="Agilent VNA", "error in (no error)"=w9, "Learn String"=w13, "VISA Resource Name"=w6) -> ("error out"=→"error out":errorcluster, "dup VISA Resource Name"=→"dup VISA Resource Name":refnum<visa-resource-name>)  [unwired: 2 in, 4 out]
